vi "Error Handler - Message Handling Loop.vi"(8 "error in (no error)":T1 caption="entrée d'erreur (pas d'erreur)", 10 "Erreurs à ignorer (exécution)":i32[](array[numeric]), 11 "File d'attente de messages":refnum<queue>) -> (0 "erreur en entrée dup.":T1, 3 "File d'attente de message dup.":refnum<queue>)   [LabVIEW 2018]
doc: "Gère une erreur qui a eu lieu dans la boucle de gestion de messages en l'ignorant ou en générant un message \"Exit\"."
uses:
  Message Queue/Message Cluster.ctl
  Message Queue/Message Queue.lvlib
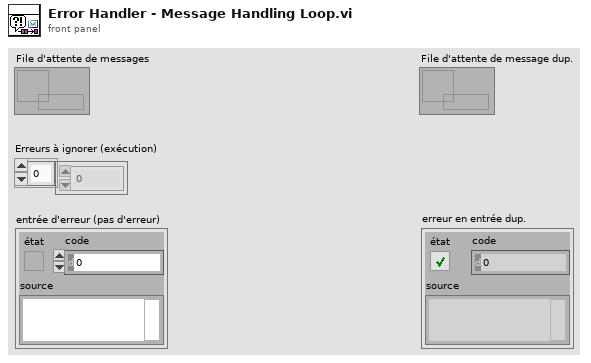
[diagram p1: front panel]
types:
  T1 = cluster{"état":bool, "code":i32, "source":string}
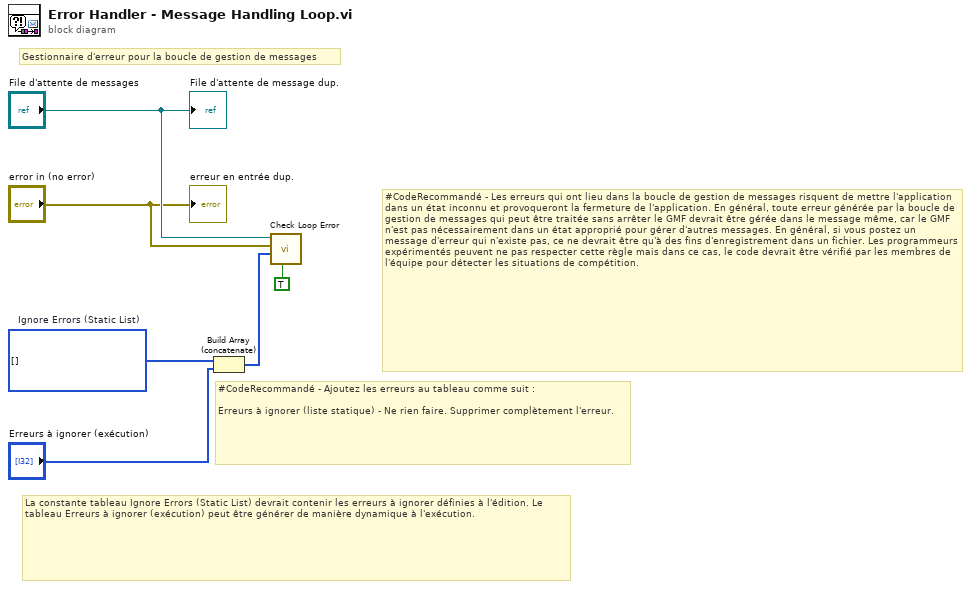
[diagram p0: block diagram]
diagram:
  w5 = i32[] []  # Ignore Errors (Static List)
  # "#CodeRecommandé - Les erreurs qui ont lieu dans la boucle de gestion de messages risquent de mettre l'application dans un état inconnu et provoqueront la fermeture de l'application. En général, toute erreur générée par la boucle de gestion de messages qui peut être traitée sans arrêter le GMF devrait être gérée dans le message même, car le GMF n'est pas nécessairement dans un état approprié pour gérer d'autres messages. En général, si vous postez un message d'erreur qui n'existe pas, ce ne devrait être qu'à des fins d'enregistrement dans un fichier. Les programmeurs expérimentés peuvent ne pas respecter cette règle mais dans ce cas, le code devrait être vérifié par les membres de l'équipe pour détecter les situations de compétition."
  # "La constante tableau Ignore Errors (Static List) devrait contenir les erreurs à ignorer définies à l'édition. Le tableau Erreurs à ignorer (exécution) peut être générer de manière dynamique à l'exécution."
  # "#CodeRecommandé - Ajoutez les erreurs au tableau comme suit :\n\nErreurs à ignorer (liste statique) - Ne rien faire. Supprimer complètement l'erreur."
  # "Gestionnaire d'erreur pour la boucle de gestion de messages"
  n1 = Build Array (concatenate)(w5, "Erreurs à ignorer (exécution)") -> (w4:i32[])
  n2 = call "Check Loop Error.vi"("Quitter en cas d'erreur ? (F)"=TRUE ("Exit on Error? (F)"), "Ignorer les erreurs"=w4, "erreur à traiter"="error in (no error)", "File d'attente de messages"="File d'attente de messages") -> ()  [unwired: 6 in, 2 out]
  "File d'attente de message dup." <- "File d'attente de messages"
  "erreur en entrée dup." <- "error in (no error)"
